vi "test Init Module.vi"(8 "error in (no error)":errorcluster, 11 "TestCase in":refnum<class "RSI Module Unit Tests.lvclass">) -> (0 "error out":errorcluster, 3 "TestCase out":refnum<class "RSI Module Unit Tests.lvclass">)   [LabVIEW 2017, in "RSI Module Unit Tests.lvclass"]
uses:
  RSI Module Unit Tests.lvclass
  RSI Module/Module Models.ctl
  RSI Module/Slot Settings.ctl
  <vilib>/addons/_JKI Toolkits/VI Tester/TestCase.llb/TestCase.lvclass
  Modules.lvlib
  RSI Module/RSI Module.lvclass
  C:/Program Files (x86)/National Instruments/LabVIEW 2017/vi.lib/addons/_JKI Toolkits/VI Tester/TestCase.llb/TestCase.lvclass
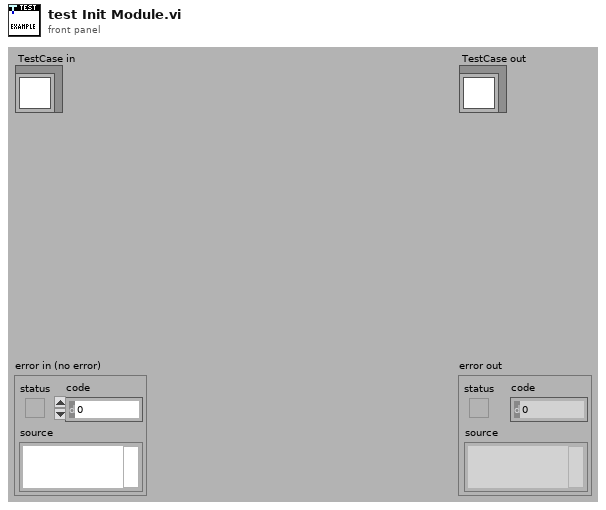
[diagram p1: front panel]
types:
  T1 = typedef "Modules.lvlib/RSI Module.lvclass/Slot Settings.ctl" = cluster{"Slot":u32, "EtherCAT?":bool}
  T2 = typedef "Modules.lvlib/RSI Module.lvclass/Module Models.ctl" = enum16{"Empty", "NI 9201", "NI 9203", "NI 9205", "NI 9206", "NI 9207", "NI 9208", "NI 9211", "NI 9212", "NI 9213", "NI 9214", "NI 9215", "NI 9217", "NI 9219", "NI 9220", "NI 9221", "NI 9222", "NI 9223", "NI 9225", "NI 9227", "NI 9229", "NI 9233", "NI 9234", "NI 9235", "NI 9236", "NI 9237", "NI 9239", "NI 9242", "NI 9244", "NI 9263", "NI 9264", "NI 9265", "NI 9266", "NI 9269", "NI 9375", "NI 9401", "NI 9402", "NI 9403", "NI 9411", "NI 9421", "NI 9422", "NI 9423", "NI 9425", "NI 9426", "NI 9435", "NI 9437", "NI 9472", "NI 9474", "NI 9475", "NI 9476", "NI 9477", "NI 9478", "NI 9481", "NI 9482", "NI 9485"}
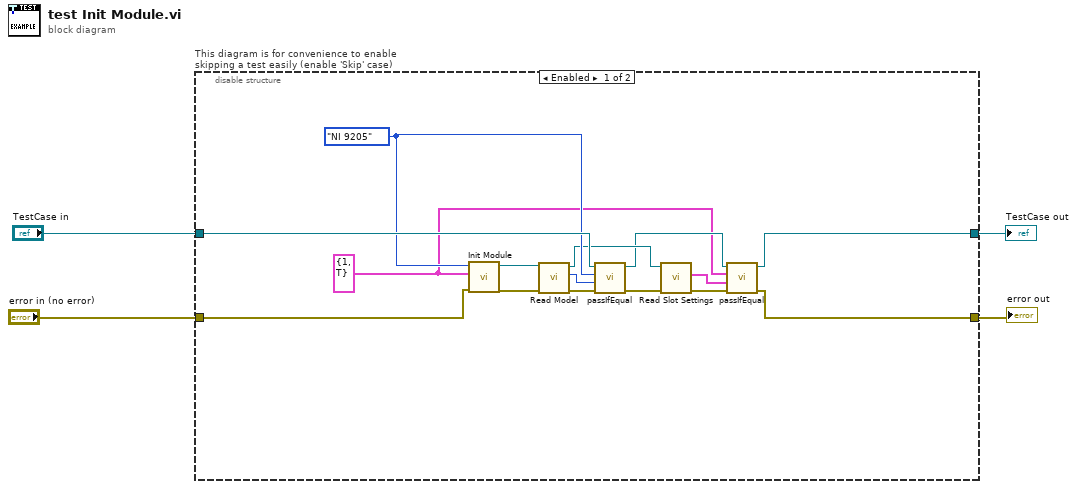
[diagram p0: block diagram]
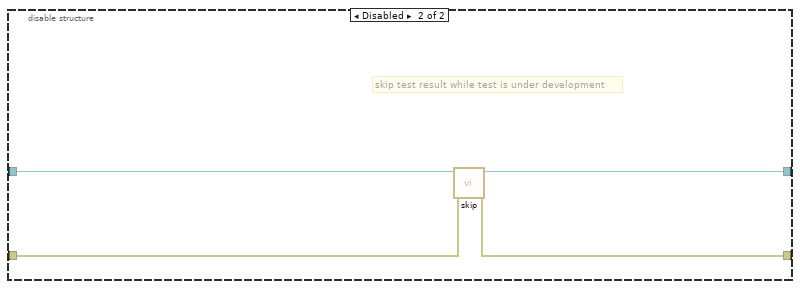
[diagram p2: hidden frame]
diagram:
  n1 = disable-structure "This diagram is for convenience to enable skipping a test easily (enable 'Skip' case)" shown="Enabled" {
    disable-tunnel: "TestCase in" -> [w19 w23]
    disable-tunnel: [w6 w21] -> w1
    disable-tunnel: [w9 w22] -> w3
    disable-tunnel: "error in (no error)" -> [w18 w20]
    frame Enabled {
      w5 = T1 {"Slot"=1, "EtherCAT?"=TRUE} ("Slot Settings")
      w15 = Module_Models."NI 9205" ("Module Model")
      n2 = call "Init Module.vi"("error in (no error)"=w18, "Slot Settings"=w5, "Module Model"=w15) -> ("error out"=w17:errorcluster, "RSI Module out"=w16:refnum<class "RSI Module.lvclass">)  [unwired: 7 in]
      n3 = call "Read Model.vi"("error in (no error)"=w17, "RSI Module in"=w16) -> ("error out"=w13:errorcluster, "Model"=w14:T2, "RSI Module out"=w11:refnum<class "RSI Module.lvclass">)  [unwired: 7 in]
      n4 = call-dynamic "passIfEqual.vi"("error in (no error)"=w13, "y"=w14, "x"=w15, "TestCase in"=w19) -> ("error out"=w12:errorcluster, "TestCase out"=w7:refnum<class "RSI Module Unit Tests.lvclass">)  [unwired: 6 in]
      n5 = call "Read Slot Settings.vi"("error in (no error)"=w12, "RSI Module in"=w11) -> ("error out"=w10:errorcluster, "Slot Settings"=w8:T1)  [unwired: 7 in, 1 out]
      n6 = call-dynamic "passIfEqual.vi"("error in (no error)"=w10, "y"=w8, "x"=w5, "TestCase in"=w7) -> ("error out"=w9:errorcluster, "TestCase out"=w6:refnum<class "RSI Module Unit Tests.lvclass">)  [unwired: 6 in]
    }
    frame Disabled {
      # "skip test result while test is under development"
      n7 = call <vilib>:"skip.vi"("error in (no error)"=w20, "TestCase in"=w23) -> ("error out"=w22:errorcluster, "TestCase out"=w21:refnum<class "RSI Module Unit Tests.lvclass">)  [unwired: 8 in]
    }
  }
  "error out" <- w3
  "TestCase out" <- w1
